vi "target motor string cluster to numeric array.vi"(1 "Target Motor Positions":T1) -> (0 "Array":dbl[](array[numeric]))   [LabVIEW 2011]
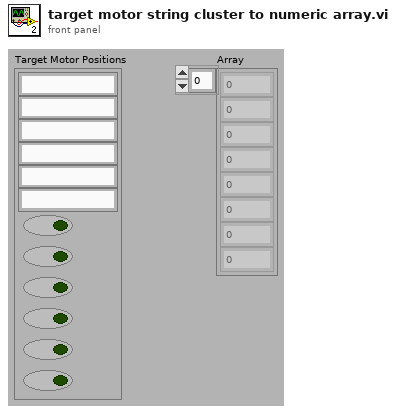
[diagram p1: front panel]
types:
  T1 = cluster{string, string, string, string, string, string, bool, bool, bool, bool, bool, bool}
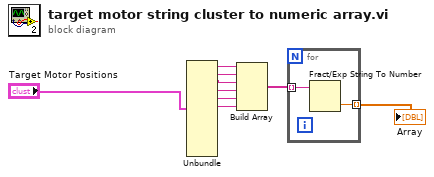
[diagram p0: block diagram]
diagram:
  n1 = Unbundle("Target Motor Positions") -> (w6:string, w5:string, w4:string, w3:string, w2:string, w1:string)  [unwired: 6 out]
  n2 = Build Array(w6, w5, w4, w3, w2, w1) -> (w8:string[])
  n3 = for {
    tunnel: w8 -> [w11] mode=indexing
    tunnel: [w10] -> w9 mode=indexing
    n4 = Fract/Exp String To Number(string=w11) -> (number=w10:dbl)  [unwired: 3 in, 1 out]
  }
  "Array" <- w9
